vi "Update State.vi"(8 "error in (no error)":errorcluster, 11 "Comp Motors with Encoders in":refnum<class "Comp Motors with Encoders.lvclass">) -> (0 "error out":errorcluster, 3 "Comp Motors with Encoders out":refnum<class "Comp Motors with Encoders.lvclass">)   [LabVIEW 2014, in "Comp Motors with Encoders.lvlib" / "Comp Motors with Encoders.lvclass"]
uses:
  Comp Motors with Encoders.lvclass
  Comp Motors with Encoders.lvclass/Comp Motors with Encoders.ctl
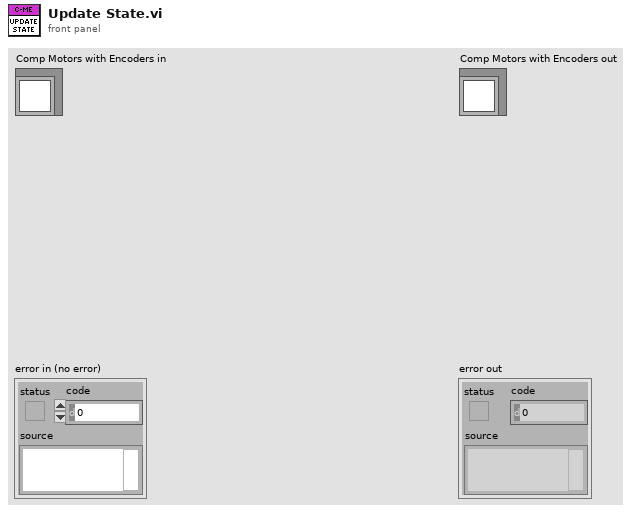
[diagram p1: front panel]
types:
  T1 = typedef "WPI_MotorControlDeviceRef.ctl" = cluster{"DeviceStatus":errorcluster, "Type":T2, "PWM":cluster{"Controller":T3, "PWM Channel":T4, "DeadBand":T5}, "CAN":cluster{"Device Number":u8, "Control Mode":T6, "Semaphore":T7, "Max Vout":dbl, "TalonSRX Control Mode":T8}, "Invert":bool, "TransformRef":T9, "InvTransformRef":T9}
  T2 = typedef "WPI_MotorControlType.ctl" = enum16{"PWM", "CAN", "CANTalonSRX"}
  T3 = typedef "FPGA_TypedefDigitalModule.ctl" = enum16{"Controller 1"}
  T4 = typedef "FPGA_DIOPWMChannel.ctl" = enum8{"PWM 0", "PWM 1", "PWM 2", "PWM 3", "PWM 4", "PWM 5", "PWM 6", "PWM 7", "PWM 8", "PWM 9", "PWM MXP 0", "PWM MXP 1", "PWM MXP 2", "PWM MXP 3", "PWM MXP 4", "PWM MXP 5", "PWM MXP 6", "PWM MXP 7", "PWM MXP 8", "PWM MXP 9", "Invalid"}
  T5 = typedef "WPI_PWMDeadband.ctl" = cluster{"Name":string, "maxPositivePwm":i32, "minPositivePwm":i32, "centerPwm":i32, "maxNegativePwm":i32, "minNegativePwm":i32, "angularRange":u16}
  T6 = typedef "WPI_CANJaguar_ControlMode.ctl" = enum8{"Percent VBus", "Current", "Speed", "Position", "Voltage"}
  T7 = typedef "Semaphore RefNum" = refnum<k1>
  T8 = typedef "WPI_CANTalonSRX_APIControlMode.ctl" = enum8{"Percent VBus", "Speed", "Position", "Slave", "Unchanged / Invalid"}
  T9 = typedef "WPI_PWMTransform_ConPane.ctl" = refnum<vi>
  T10 = typedef "WPI_CANTalonSRX_GlobalStatus.ctl" = cluster{"Applied Throttle":dbl, "Module Enabled":bool, "CAN Error":errorcluster, "Closed Loop Error":dbl, "Forward Limit Switch Closed":bool, "Reverse Limit Switch Closed":bool, "Sensor Position":dbl, "Sensor Velocity":dbl, "Current":dbl, "Sticky Fault - Over Temp":bool, "Sticky Fault - Under Voltage":bool, "Sticky Fault - Forward Limit":bool, "Sticky Fault - Reverse Limit":bool, "Sticky Fault - Forward Soft Limit":bool, "Sticky Fault - Reverse Soft Limit":bool, "Brake is Enabled":bool, "Encoder Position":dbl, "Encoder Velocity":dbl, "Encoder Index Count":dbl, "Encoder A Pin State":bool, "Encoder B Pin State":bool, "Encoder Index Pin State":bool, "Analog In":dbl, "Analog In Velocity":dbl, "Temperature (C)":dbl, "Battery Voltage":dbl}
  T11 = typedef "Motors with Encoders.lvlib/Motors with Encoders.lvclass/Motors with Encoders State.ctl" = cluster{"Forward Switch":bool, "Reverse Switch":bool, "Measured RPM":dbl, "Distance (in)":dbl, "Setpoint RPM":dbl, "Encoder Count":i64, "Home Count":i64, "Config":T12}
  T12 = typedef "Motors with Encoders.lvlib/Motors with Encoders.lvclass/Motors with Encoders Config.ctl" = cluster{"Counts  Per Revolution":u32, "Invert Encoder Direction":bool, "Diameter of Revolution":dbl, "Max RPM":dbl, "Encoder Control":bool}
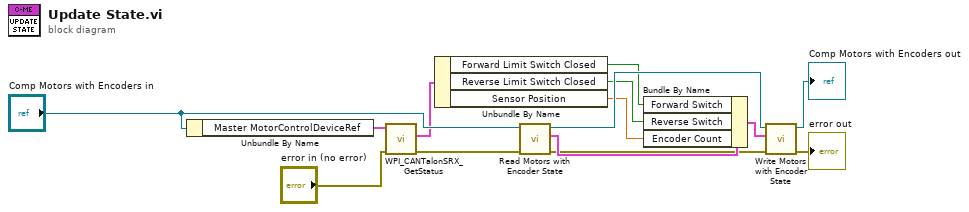
[diagram p0: block diagram]
diagram:
  n1 = Unbundle By Name("Comp Motors with Encoders in") -> ("Master MotorControlDeviceRef"=w14:T1)
  n2 = call <vilib>:"WPI_CANTalonSRX_GetStatus.vi"("error in (no error)"="error in (no error)", "CAN Talon SRX Ref"=w14) -> ("error out"=w3:errorcluster, "Talon SRX Status"=w10:T10)  [unwired: 7 in, 1 out]
  n3 = Unbundle By Name(w10) -> ("Forward Limit Switch Closed"=w7:bool, "Reverse Limit Switch Closed"=w6:bool, "Sensor Position"=w5:dbl)
  n4 = call-dynamic "Read Motors with Encoder State.vi"("error in (no error)"=w3, "Motors with Encoders in"="Comp Motors with Encoders in") -> ("error out"=w2:errorcluster, "Motors with Encoder State"=w9:T11, "Motors with Encoders out"=w13:refnum<class "Comp Motors with Encoders.lvclass">)  [unwired: 7 in]
  n5 = Bundle By Name(cluster=w9, "Forward Switch"=w7, "Reverse Switch"=w6, "Encoder Count"=w5) -> (w8:T11)
  n6 = call-dynamic "Write Motors with Encoder State.vi"("error in (no error)"=w2, "Motors with Encoder State"=w8, "Motors with Encoders in"=w13) -> ("error out"=→"error out":errorcluster, "Motors with Encoders out"=→"Comp Motors with Encoders out":refnum<class "Comp Motors with Encoders.lvclass">)  [unwired: 7 in]
